vi "__New GoL__.vi"(8 "error in":errorcluster, 9 "Pixel Size":i16=1, 10 "Grid":u8[][](array[numeric]), 11 "GoL in":refnum<class "GoL.lvclass">) -> (0 "error out":errorcluster, 3 "GoL out":refnum<class "GoL.lvclass">)   [LabVIEW 2026, in "GoL.lvlib" / "GoL.lvclass"]
uses:
  GoL.lvclass
  GoL.lvclass/GoL.ctl
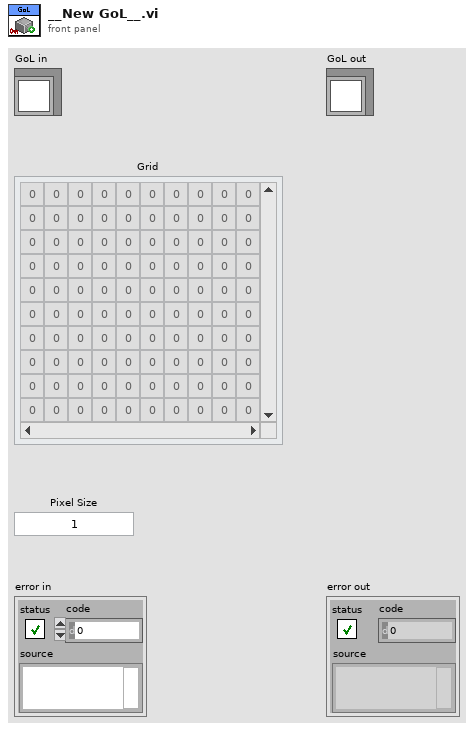
[diagram p1: front panel]
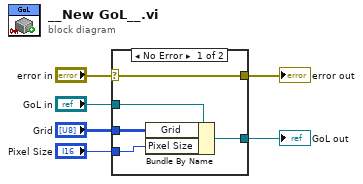
[diagram p0: block diagram]
diagram:
  n1 = case shown="No Error" "error in" {
    selector: "error in" -> [w11 w13]
    tunnel: [w11 w13] -> w5
    tunnel: [w8 w12] -> w3
    tunnel: "GoL in" -> [w10 w12]
    tunnel: "Grid" -> [w9 _]
    tunnel: "Pixel Size" -> [w7 _]
    frame No Error {
      n2 = Bundle By Name(cluster=w10, "Grid"=w9, "Pixel Size"=w7) -> (w8:refnum<class "GoL.lvclass">)
    }
    frame Error {
    }
  }
  "error out" <- w5
  "GoL out" <- w3
